vi "LV to ITX 2.2 XY.vi"(0 "Commands":string, 5 "filename":path, 7 "Notes":string, 8 "wavenames":string[](array[string]), 9 "XY Array":cluster{"X  array":dbl[], "Y  Array":dbl[]}[](array[cluster])) -> (3 "file":path)   [LabVIEW 2011]
panel:
  out "String":string
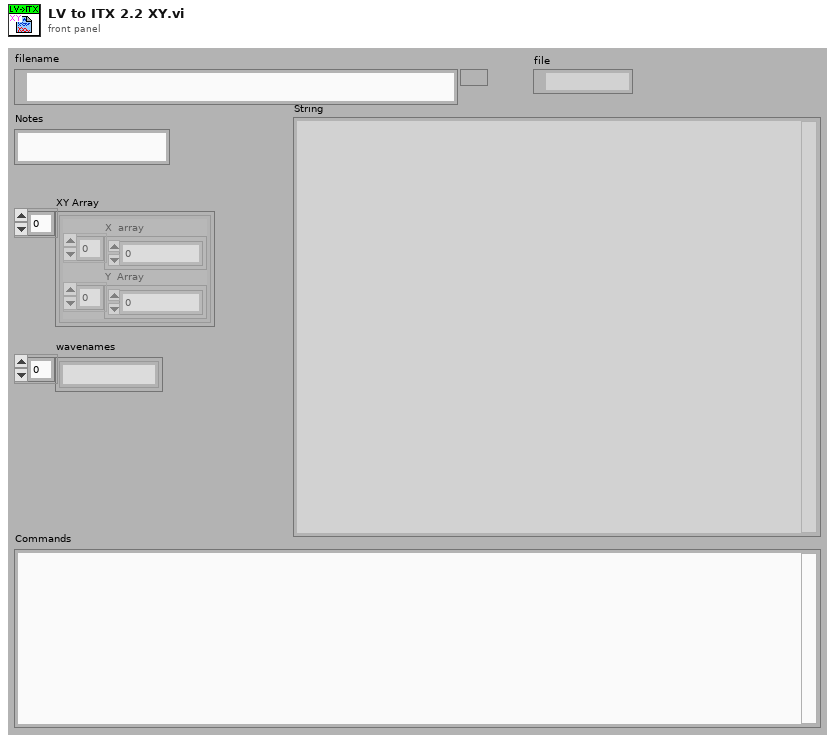
[diagram p1: front panel]
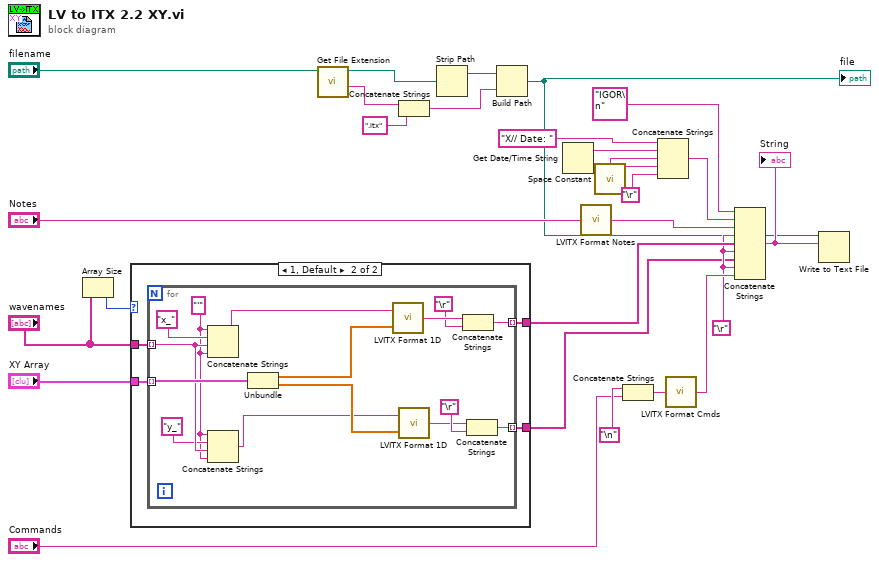
[diagram p0: block diagram]
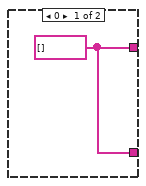
[diagram p2: hidden frame]
diagram:
  w6 = "\r"
  n1 = Array Size(array="wavenames") -> (size(s)=w12:i32)
  n2 = case shown="1, Default" w12 {
    tunnel: "wavenames" -> [_ w32]
    tunnel: "XY Array" -> [_ w31]
    tunnel: [w28 w30] -> w15
    tunnel: [w28 w29] -> w5
    frame 0 {
      w28 = string[] []
    }
    frame 1, Default {
      n3 = for {
        tunnel: [w47] -> w30 mode=indexing
        tunnel: w32 -> [w43] mode=indexing
        tunnel: w31 -> [w44] mode=indexing
        tunnel: [w36] -> w29 mode=indexing
        w35 = "'"
        n4 = Concatenate Strings(w35, "x_", w43, w35) -> (w34:string)
        n5 = Concatenate Strings(w35, "y_", w43, w35) -> (w33:string)
        n6 = Unbundle(w44) -> ("X  array"=w38:dbl[], "Y  Array"=w37:dbl[])
        n7 = call "LVITX Format 1D.vi"("X 1D Array"=w38, "X  Array name"=w34) -> ("String"=w46:string)
        n8 = call "LVITX Format 1D.vi"("X 1D Array"=w37, "X  Array name"=w33) -> ("String"=w39:string)
        n9 = Concatenate Strings(w46, "\r") -> (w47:string)
        n10 = Concatenate Strings(w39, "\r") -> (w36:string)
      }
    }
  }
  n11 = call <vilib>:"Get File Extension.vi"("file"="filename") -> ("filename without extension"=w22:string, "dup file"=w19:path)  [unwired: 1 in, 8 out]
  n12 = Concatenate Strings(w22, ".itx") -> (w17:string)
  n13 = Strip Path(path=w19) -> (stripped path=w18:path)  [unwired: 1 out]
  n14 = Build Path(base path=w18, name or relative path=w17) -> (appended path=w1:path)
  "file" <- w1
  n15 = Get Date/Time String() -> (date string=w26:string, time string=w27:string)  [unwired: 3 out]
  n16 = call "LVITX Format Notes.vi"("Notes"="Notes") -> ("String"=w2:string)
  n17 = call <vilib>:"Space Constant.vi"() -> ("String"=w24:string)
  n18 = Concatenate Strings("\n", "Commands") -> (w20:string)
  n19 = Concatenate Strings("X// Date: " ("format string"), w26, w24, w27, "\r") -> (w4:string)
  n20 = call "LVITX Format Cmds.vi"("Commands"=w20) -> ("String"=w7:string)
  n21 = Concatenate Strings("IGOR\n", w4, w2, w6, w15, w6, w5, w6, w7) -> (w14:string)
  "String" <- w14
  n22 = Write to Text File(file (use dialog)=w1, text=w14) -> ()  [unwired: 1 in, 4 out]
